vi "line to strings.vi"(11 "line":T1) -> (3 "strings":string[](array[string]))   [LabVIEW 2013, in "Profibus Module editor node.lvclass"]
uses:
  Profibus Module editor node.lvclass
  table line.ctl
  channel/Profibus channel.lvclass
  <vilib>/NI/Tag Bus/tag/tag descriptor.lvclass/tag descriptor.ctl
  channel/Profibus channel.lvclass/Profibus channel.ctl
  <vilib>/NI/Tag Bus Module Framework/channel/TBM channel.lvclass/TBM channel.ctl
  <vilib>/NI/Tag Bus/tag/read tag name.vi
  channel/Read slave.vi
  channel/Read byte.vi
  channel/Read bit.vi
  <vilib>/NI/Tag Bus Module Framework/channel/Read channel classification.vi
  <vilib>/NI/Tag Bus/tag/read data type.vi
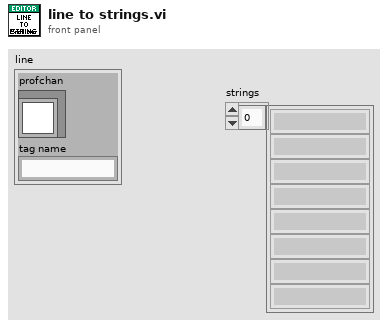
[diagram p1: front panel]
types:
  T1 = typedef "Profibus Module editor node.lvclass/table line.ctl" = cluster{"profchan":refnum<class "Profibus channel.lvclass">, "tag name":string}
  T2 = typedef "TBM channel.lvclass/channel classification.ctl" = enum16{"input data", "output data", "processing parameter", "processing result"}
  T3 = typedef "tag bus.lvlib/tag descriptor.lvclass/Data Type.ctl" = enum16{"Double", "Single", "I64", "I32", "I16", "I8", "U64", "U32", "U16", "U8", "Boolean", "String", "Array of Double", "Array of Single", "Array of I64", "Array of I32", "Array of I16", "Array of I8", "Array of U64", "Array of U32", "Array of U16", "Array of U8", "Array of Boolean", "Array of String"}
  T4 = typedef "Profibus Module editor node.lvclass/permissions.ctl" = enum32{"Read from HW", "Write to HW"}
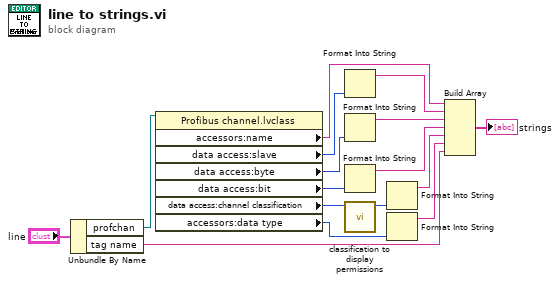
[diagram p0: block diagram]
diagram:
  n1 = Unbundle By Name("line") -> ("profchan"=w10:refnum<class "Profibus channel.lvclass">, "tag name"=w14:string)
  n2 = property class="Profibus channel.lvclass"(reference=w10) -> ("accessors:name"=w7:string, "data access:slave"=w1:i8, "data access:byte"=w2:i32, "data access:bit"=w3:i32, "data access:channel classification"=w9:T2, "accessors:data type"=w8:T3)  [unwired: 1 in, 2 out]
  n3 = Format Into String(w1) -> (resulting string=w6:string)  [unwired: 3 in, 1 out]
  n4 = Format Into String(w2) -> (resulting string=w5:string)  [unwired: 3 in, 1 out]
  n5 = Format Into String(w3) -> (resulting string=w4:string)  [unwired: 3 in, 1 out]
  n6 = call "classification to display permissions.vi"("channel classification"=w9) -> ("permissions"=w12:T4)  [unwired: 10 in]
  n7 = Format Into String(w12) -> (resulting string=w11:string)  [unwired: 3 in, 1 out]
  n8 = Format Into String(w8) -> (resulting string=w15:string)  [unwired: 3 in, 1 out]
  n9 = Build Array(w7, w6, w5, w4, w11, w15, w14) -> (→"strings":string[])
